vi "Negative Feedback with Rational Polynomials (CDB).vi"(8 "Denominator 2":cdb[](array[numeric]) format="%#.2g", 9 "Numerator 2":cdb[](array[numeric]) format="%#.2g", 10 "Denominator 1":cdb[](array[numeric]) format="%#.2g", 11 "Numerator 1":cdb[](array[numeric]) format="%#.2g") -> (0 "error":i32, 2 "Denominator Out":cdb[](array[numeric]) format="%#.2g", 3 "Numerator Out":cdb[](array[numeric]) format="%#.2g")   [LabVIEW 2020, in "NI_AALPro.lvlib"]
doc: "Calculates the negative feedback equation. The data types you wire to the <B>Numerator 1</B>, <B>Denominator 1</B>, <B>Numerator 2</B>, and <B>Denominator 2</B> inputs determine the polymorphic instance to use."
uses:
  NI_AALPro.lvlib
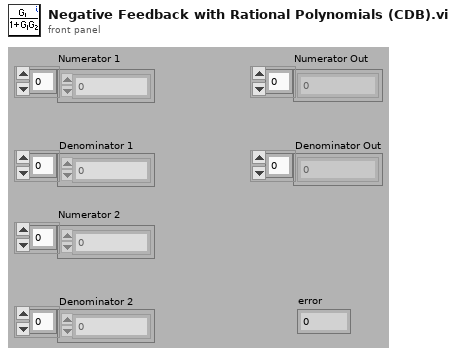
[diagram p1: front panel]
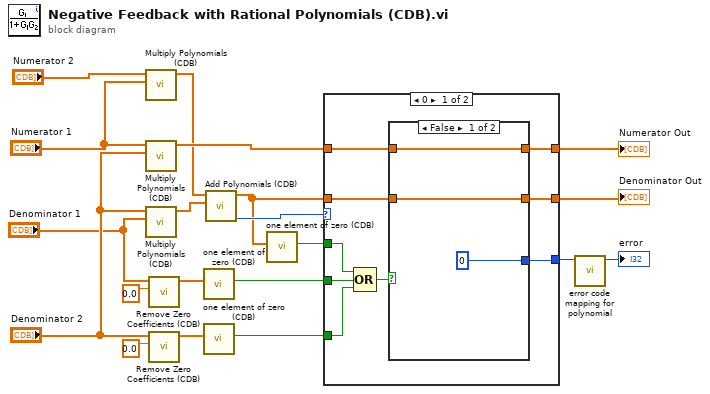
[diagram p0: block diagram]
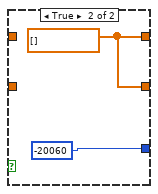
[diagram p2: hidden frame]
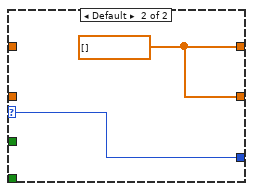
[diagram p3: hidden frame]
diagram:
  n1 = call "Multiply Polynomials (CDB).vi"("Q(x)"="Numerator 1", "P(x)"="Numerator 2") -> ("P(x)*Q(x)"=w11:cdb[])  [unwired: 8 in, 1 out]
  n2 = call "Multiply Polynomials (CDB).vi"("Q(x)"="Denominator 2", "P(x)"="Numerator 1") -> ("P(x)*Q(x)"=w18:cdb[])  [unwired: 8 in, 1 out]
  n3 = call "Multiply Polynomials (CDB).vi"("Q(x)"="Denominator 1", "P(x)"="Denominator 2") -> ("P(x)*Q(x)"=w12:cdb[])  [unwired: 8 in, 1 out]
  n4 = call "Remove Zero Coefficients (CDB).vi"("threshold"=0.0, "P(x) In"="Denominator 1") -> ("P(x) Out"=w8:cdb[])  [unwired: 7 in, 2 out]
  n5 = call "Remove Zero Coefficients (CDB).vi"("threshold"=0.0, "P(x) In"="Denominator 2") -> ("P(x) Out"=w15:cdb[])  [unwired: 7 in, 2 out]
  n6 = call "one element of zero (CDB).vi"("Array in"=w8) -> ("equal [0]?"=w6:bool)  [unwired: 10 in]
  n7 = call "one element of zero (CDB).vi"("Array in"=w15) -> ("equal [0]?"=w5:bool)  [unwired: 10 in]
  n8 = call "Add Polynomials (CDB).vi"("Q(x)"=w12, "P(x)"=w11) -> ("error"=w17:i32, "P(x)+Q(x)"=w4:cdb[])  [unwired: 8 in]
  n9 = call "one element of zero (CDB).vi"("Array in"=w4) -> ("equal [0]?"=w3:bool)  [unwired: 10 in]
  n10 = case shown="0" w17 {
    selector: w17 -> [_ w35]
    tunnel: w18 -> [w28 _]
    tunnel: w4 -> [w29 _]
    tunnel: [w27 w36] -> w20
    tunnel: [w26 w36] -> w19
    tunnel: [w25 w35] -> w2
    tunnel: w6 -> [w23 _]
    tunnel: w5 -> [w24 _]
    tunnel: w3 -> [w21 _]
    frame 0 {
      n11 = Compound Arithmetic op=OR(w21, w23, w24) -> (w22:bool)
      n12 = case shown="False" w22 {
        tunnel: [0 -20060 ("divide by zero")] -> w25
        tunnel: w29 -> [w31 _]
        tunnel: w28 -> [w32 _]
        tunnel: [w32 w34] -> w27
        tunnel: [w31 w34] -> w26
        frame False {
        }
        frame True {
          w34 = cdb[] [] ("CDB")
        }
      }
    }
    frame Default {
      w36 = cdb[] [] ("CDB")
    }
  }
  "Numerator Out" <- w20
  "Denominator Out" <- w19
  n13 = call "error code mapping for polynomial.vi"("error in"=w2) -> ("error out"=→"error":i32)  [unwired: 10 in]
